vi "StopAsyncWorker.vi"(8 "error in (no error)":errorcluster, 10 "WaitOnAsync?":bool, 11 "ResultProcessor in":refnum<class "ResultProcessor.lvclass">) -> (0 "error out":errorcluster, 3 "ResultProcessor out":refnum<class "ResultProcessor.lvclass">)   [LabVIEW 2015, in "ResultProcessor.lvclass"]
doc: "This VI will enqueue a shutdown command for the async worker. If <b>WaitOnAsync?</b> is True, it will wait for the worker to shutdown before exiting. The timeout for this wait is 100 seconds."
uses:
  ResultProcessor.lvclass
  CommandQueueDataType.ctl
  Report Information/Report Information.lvclass
  Result/Result.lvclass
  ResultProcessor.lvclass/ResultProcessor.ctl
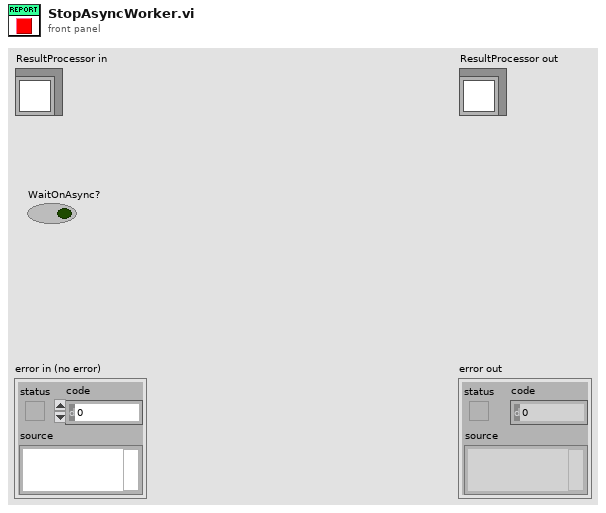
[diagram p1: front panel]
types:
  T1 = typedef "ResultProcessor.lvclass/CommandQueueDataType.ctl" = cluster{"Command":enum16{"New Report", "Add Result", "Publish Report", "Shutdown", "Add DUT Information", "Add Station Information", "Add Report Information", "Add Test Information"}, "Report Information.lvclass":refnum<class "Report Information.lvclass">, "Result.lvclass":refnum<class "Result.lvclass">}
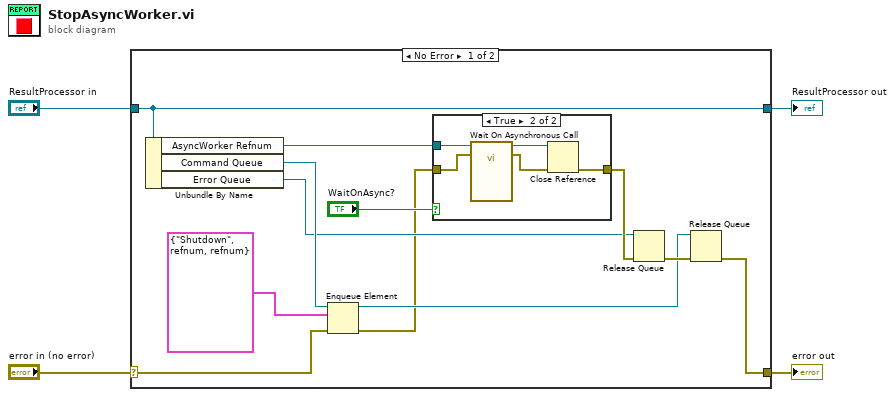
[diagram p0: block diagram]
diagram:
  n1 = case shown="No Error" "error in (no error)" {
    selector: "error in (no error)" -> [w14 w24]
    tunnel: [w9 w24] -> w3
    tunnel: [w16 w23] -> w1
    tunnel: "ResultProcessor in" -> [w16 w23]
    frame No Error {
      n2 = Unbundle By Name(w16) -> ("AsyncWorker Refnum"=w5:refnum<vi>, "Command Queue"=w15:refnum<queue>, "Error Queue"=w7:refnum<queue>)
      n3 = Enqueue Element(queue=w15, element=T1 {"Command"=enum."Shutdown", "Report Information.lvclass"=refnum, "Result.lvclass"=refnum}, error in (no error)=w14) -> (queue out=w8:refnum<queue>, error out=w6:errorcluster)  [unwired: 1 in, 1 out]
      n4 = case shown="True" "WaitOnAsync?" {
        tunnel: w5 -> [_ w22]
        tunnel: [w17 w19] -> w12
        tunnel: w6 -> [w17 w18]
        frame False {
        }
        frame True {
          n5 = call-by-ref "Wait On Asynchronous Call"(reference=w22, error in=w18) -> (reference out=w21:refnum<vi>, error out=w20:errorcluster)  [unwired: 12 in]
          n6 = Close Reference(reference=w21, error in (no error)=w20) -> (error out=w19:errorcluster)
        }
      }
      n7 = Release Queue(queue=w7, error in (no error)=w12) -> (error out=w10:errorcluster)  [unwired: 1 in, 2 out]
      n8 = Release Queue(queue=w8, error in (no error)=w10) -> (error out=w9:errorcluster)  [unwired: 1 in, 2 out]
    }
    frame Error {
    }
  }
  "error out" <- w3
  "ResultProcessor out" <- w1
